vi "Read Initial Frequency and Phase.vi"(8 "error in (no error)":errorcluster, 11 "SV Continuous Sweep in":refnum<class "SV Continuous Sweep.lvclass">) -> (0 "error out":errorcluster, 1 "initial phase":dbl, 2 "initial frequency":dbl, 3 "SV Continuous Sweep out":refnum<class "SV Continuous Sweep.lvclass">, 4 "found?":bool)   [LabVIEW 2017, in "SV Continuous Sweep.lvclass"]
uses:
  <vilib>/addons/_NISVFA/_Generation/Signal Generation/SV Continuous Sweep/SV Continuous Sweep.lvclass
  <vilib>/addons/_NISVFA/_Generation/Signal Generation/SV Continuous Sweep/SV Continuous Sweep.lvclass/SV Continuous Sweep.ctl
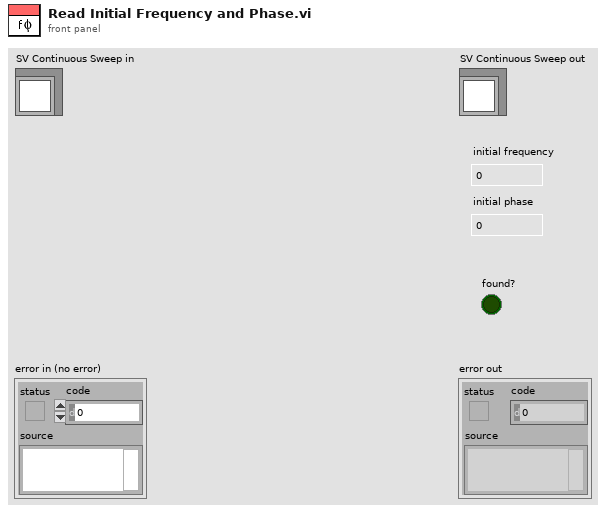
[diagram p1: front panel]
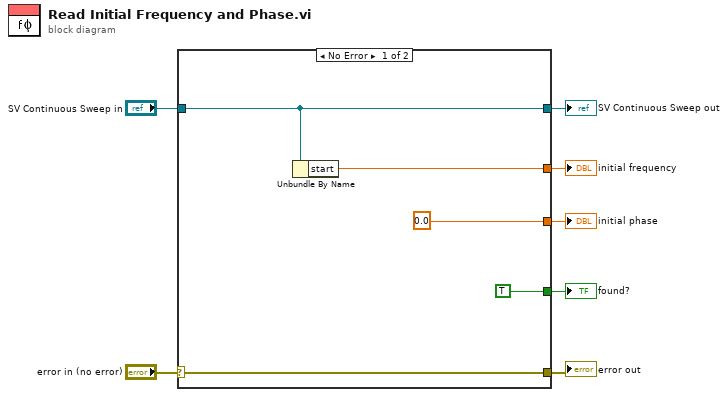
[diagram p0: block diagram]
diagram:
  n1 = case shown="No Error" "error in (no error)" {
    selector: "error in (no error)" -> [w12 w14]
    tunnel: [w12 w14] -> w2
    tunnel: [w10 w13] -> w5
    tunnel: "SV Continuous Sweep in" -> [w10 w13]
    tunnel: [TRUE ("found?") _] -> w1
    tunnel: [0.0 ("duration [s]") _] -> w4
    tunnel: [w9 _] -> w3
    frame No Error {
      n2 = Unbundle By Name(w10) -> ("start"=w9:dbl)
    }
    frame Error {
    }
  }
  "error out" <- w2
  "SV Continuous Sweep out" <- w5
  "initial frequency" <- w3
  "initial phase" <- w4
  "found?" <- w1
